vi "UDP Begin Packet IP Test.vi"() -> ()   [LabVIEW 2014, in "ESP8266 WiFi Wrapper.lvlib"]
uses:
  <vilib>/Aledyne-TSXperts/Arduino Compatible Compiler for LabVIEW/addons/ESP8266 WiFi Wrapper/ESP8266 WiFi Wrapper.lvlib
panel:
  in  "IP Address":u8[](array[numeric])=[127, 0, 0, 1]
  in  "Port":u8=74
  out "Successful?":bool
  out "Error Out":errorcluster
  in  "Error In":errorcluster
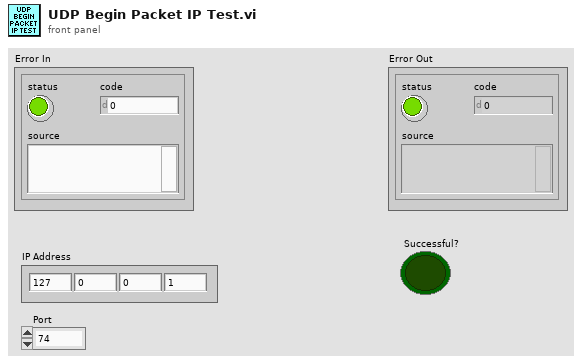
[diagram p1: front panel]
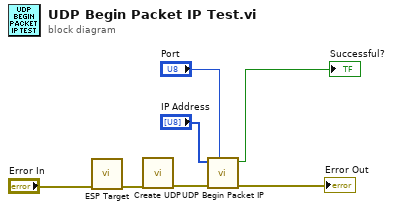
[diagram p0: block diagram]
diagram:
  n1 = call <vilib>:"ESP Target.vi"("Error In"="Error In") -> ("Error Out"=w6:errorcluster)  [unwired: 10 in]
  n2 = call <vilib>:"Create UDP.vi"("Error In"=w6) -> ("Error Out"=w5:errorcluster)  [unwired: 10 in]
  n3 = call <vilib>:"UDP Begin Packet IP.vi"("Port"="Port", "Error In"=w5, "IP Address"="IP Address") -> ("Error Out"=→"Error Out":errorcluster, "Successful?"=→"Successful?":bool)  [unwired: 7 in]
